vi "GetInstance.vi"(5 "error in (no error)":errorcluster) -> (14 "reference out":refnum<class "SingletonTemplate.lvclass">, 19 "error out":errorcluster)   [LabVIEW 2020, in "SingletonTemplate.lvclass"]
uses:
  <resource>/Framework/Providers/Open_GDS/ClassProviders/Provider_EndevoGOOP300/Templates/SingletonTemplate/SingletonTemplate.lvclass
panel:
  in  "DummyRef(hidden)":refnum<class "SingletonTemplate.lvclass">
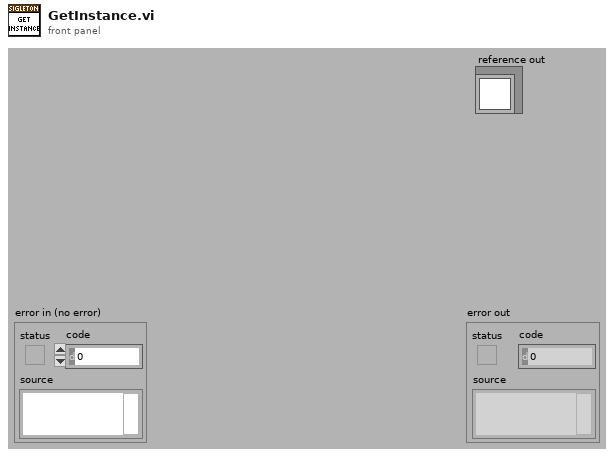
[diagram p1: front panel]
types:
  T1 = enum16{"Create", "Create or look up existing", "Look up existing"}
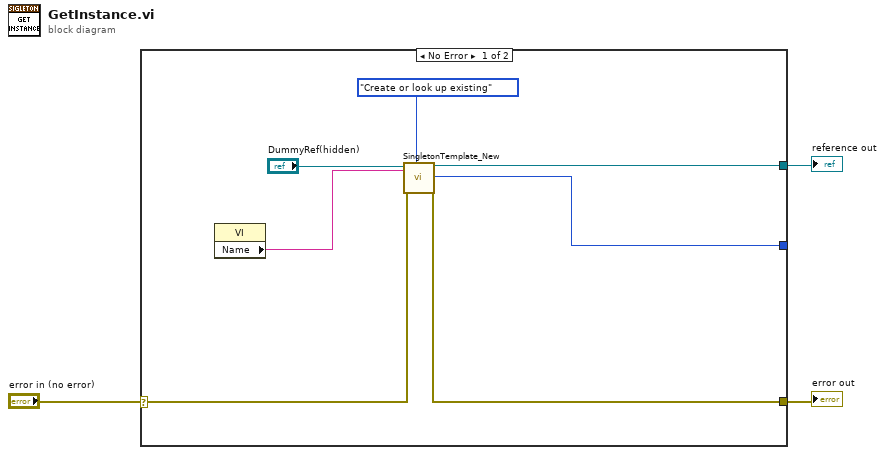
[diagram p0: block diagram]
diagram:
  n1 = case shown="No Error" "error in (no error)" {
    selector: "error in (no error)" -> [w10 w11]
    tunnel: [w9 w11] -> w3
    tunnel: [w8 _] -> w1
    tunnel: [w4 _] -> _
    frame No Error {
      n2 = property class="VI"() -> ("Name"=w5:string)  [unwired: 2 in, 2 out]
      n3 = call <resource>:"SingletonTemplate_New.vi"("reference in"="DummyRef(hidden)", "Object name"=w5, "error in (no error)"=w10, "Create method"=T1."Create or look up existing") -> ("reference out"=w8:refnum<class "SingletonTemplate.lvclass">, "# of objects"=w4:i32, "error out"=w9:errorcluster)  [unwired: 12 in, 1 out]
    }
    frame Error {
    }
  }
  "error out" <- w3
  "reference out" <- w1
